vi "FileIoManager.vi"(8 "error in":errorcluster, 9 "slmDataSetIn":T1={"BeamParameters"={"amplitudeMatrix"=[], "SLM width (m)"=0.01536, "SLM height (m)"=0.00864, "wavelength (m)"=6.33e-07, "Resolution x"=1920, "Resolution y"=1080}, "BeamControl"={"xCenter"=0.0, "yCenter"=0.0, "xAngle_mRad"=4.5, "yAngle_mRad"=0.0, "beamWaist"=0.001}, "SLM Settings"={"resizeTo"=enum."Width of Display", "displayOn"=enum."All 2nd Monitor", "Top Left of Hologram"={"Horizontal"=80, "Vertical"=80}}, "Gamma Function"=245.0, "SLM colour coding"=enum."8-bit", "Masking?"=TRUE, "Calibration?"=FALSE, "Modes"=[{"type"=enum."LG Mode", "m or L"=2, "n or P"=0, "weight"=1.0, "phase"=0.0}, {"type"=enum."LG Mode", "m or L"=-2, "n or P"=0, "weight"=1.0, "phase"=0.0}, {"type"=enum."LG Mode", "m or L"=0, "n or P"=0, "weight"=0.0, "phase"=0.0}, {"type"=enum."LG Mode", "m or L"=0, "n or P"=0, "weight"=0.0, "phase"=0.0}], "Holo"=enum."Show", "BMP filePath"=path "C:/Users/science/Desktop/Filippo The 2nd/LabVIEW/Holos/SLMA/HG_2_2.bmp", "Power Meter Settings"={"Visa In"="", "Averaging Rate"=300, "Graph Length"=1000}, "Flip Image"=FALSE, "Mirror image"=FALSE, "Phase rotation"=0.0} {"Phase rotation" min=-6.2832 max=6.28318530718 step=0.01570796326; "BeamParameters"."Resolution y" format="%#.4g"; "BeamParameters"."Resolution x" format="%#.6g"}, 10 "file (use dialog)":path, 11 "state":enum16{"read", "write"}(ring)) -> (0 "error out":errorcluster, 1 "slmDataSetOut":T1={"BeamParameters"={"amplitudeMatrix"=[], "SLM width (m)"=0.01536, "SLM height (m)"=0.00864, "wavelength (m)"=6.33e-07, "Resolution x"=1920, "Resolution y"=1080}, "BeamControl"={"xCenter"=0.0, "yCenter"=0.0, "xAngle_mRad"=4.5, "yAngle_mRad"=0.0, "beamWaist"=0.001}, "SLM Settings"={"resizeTo"=enum."Width of Display", "displayOn"=enum."All 2nd Monitor", "Top Left of Hologram"={"Horizontal"=80, "Vertical"=80}}, "Gamma Function"=245.0, "SLM colour coding"=enum."8-bit", "Masking?"=TRUE, "Calibration?"=FALSE, "Modes"=[{"type"=enum."LG Mode", "m or L"=2, "n or P"=0, "weight"=1.0, "phase"=0.0}, {"type"=enum."LG Mode", "m or L"=-2, "n or P"=0, "weight"=1.0, "phase"=0.0}, {"type"=enum."LG Mode", "m or L"=0, "n or P"=0, "weight"=0.0, "phase"=0.0}, {"type"=enum."LG Mode", "m or L"=0, "n or P"=0, "weight"=0.0, "phase"=0.0}], "Holo"=enum."Show", "BMP filePath"=path "C:/Users/science/Desktop/Filippo The 2nd/LabVIEW/Holos/SLMA/HG_2_2.bmp", "Power Meter Settings"={"Visa In"="", "Averaging Rate"=300, "Graph Length"=1000}, "Flip Image"=FALSE, "Mirror image"=FALSE, "Phase rotation"=0.0} {"Phase rotation" min=-6.2832 max=6.28318530718 step=0.01570796326; "BeamParameters"."Resolution y" format="%#.4g"; "BeamParameters"."Resolution x" format="%#.6g"})   [LabVIEW 2020]
uses:
  typeDefs/fileIO.ctl
  typeDefs/BPandSLM.ctl
  typeDefs/beamData.ctl
  typeDefs/slmSettings.ctl
  typeDefs/modesArray.ctl
  typeDefs/modeCluster.ctl
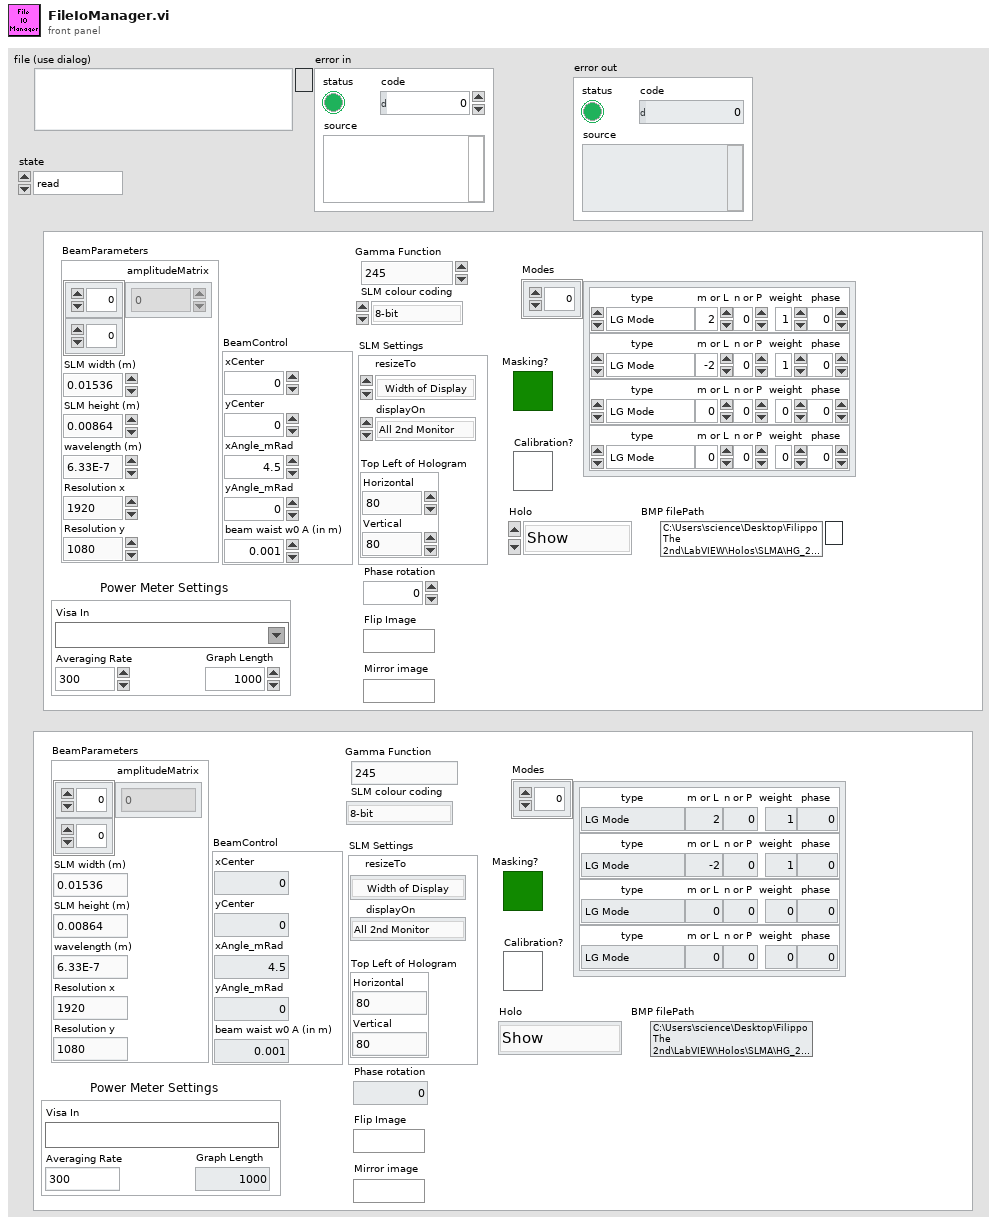
[diagram p1: front panel]
types:
  T1 = typedef "fileIO.ctl" = cluster{"BeamParameters":T2, "BeamControl":T3, "SLM Settings":T4, "Gamma Function":dbl, "SLM colour coding":enum16{"8-bit", "10-bit (Santec)"}, "Masking?":bool, "Calibration?":bool, "Modes":T5, "Holo":enum16{"Show", "Save BMP"}, "BMP filePath":path, "Power Meter Settings":cluster{"Visa In":refnum<visa-resource-name>, "Averaging Rate":i32, "Graph Length":i32}, "Flip Image":bool, "Mirror image":bool, "Phase rotation":dbl}
  T2 = typedef "BPandSLM.ctl" = cluster{"amplitudeMatrix":csg[][], "SLM width (m)":dbl, "SLM height (m)":dbl, "wavelength (m)":dbl, "Resolution x":u32, "Resolution y":u32}
  T3 = typedef "beamData.ctl" = cluster{"xCenter":dbl, "yCenter":dbl, "xAngle_mRad":dbl, "yAngle_mRad":dbl, "beamWaist":dbl}
  T4 = typedef "slmSettings.ctl" = cluster{"resizeTo":enum16{"No Resize", "Width of Display", "Height of Display"}, "displayOn":enum16{"Default", "All 1st Monitor", "All 2nd Monitor", "All 3rd Monitor", "All 4th Monitor"}, "Top Left of Hologram":cluster{"Horizontal":i16, "Vertical":i16}}
  T5 = typedef "modesArray.ctl" = T6[]
  T6 = typedef "modeCluster.ctl" = cluster{"type":enum16{"Azimuth Mode", "LG Mode", "HG Mode"}, "m or L":i32, "n or P":i32, "weight":dbl, "phase":dbl}
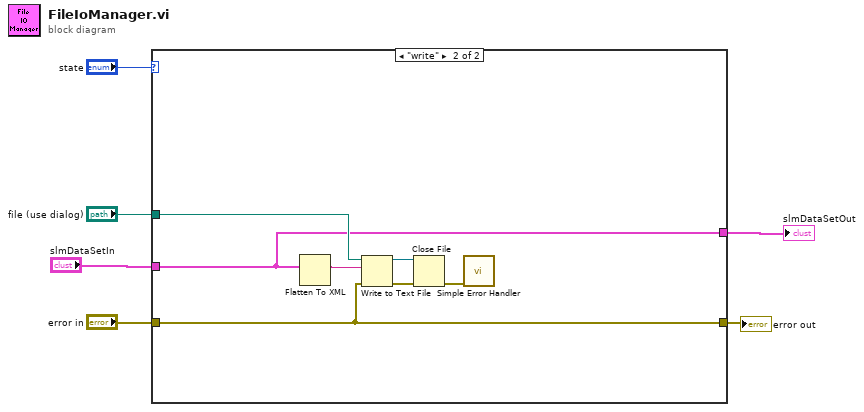
[diagram p0: block diagram]
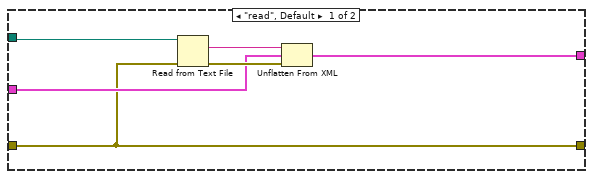
[diagram p2: hidden frame]
diagram:
  n1 = case shown="\"write\"" "state" {
    tunnel: "file (use dialog)" -> [w12 w18]
    tunnel: "error in" -> [w7 w14]
    tunnel: [w7 w14] -> w3
    tunnel: "slmDataSetIn" -> [w9 w13]
    tunnel: [w8 w13] -> w2
    frame "read", Default {
      n2 = Read from Text File(file (use dialog)=w12, error in=w7) -> (text=w11:string, error out=w10:errorcluster)  [unwired: 2 in, 2 out]
      n3 = Unflatten From XML(xml string=w11, type=w9, error in (no error)=w10) -> (value=w8:T1)  [unwired: 1 out]
    }
    frame "write" {
      n4 = Flatten To XML(6:w13) -> (2:w19:string)
      n5 = Write to Text File(file (use dialog)=w18, text=w19, error in=w14) -> (refnum out=w16:refnum<file>, error out=w17:errorcluster)  [unwired: 1 in, 1 out]
      n6 = Close File(refnum=w16, error in=w17) -> (error out=w15:errorcluster)  [unwired: 1 out]
      n7 = call <vilib>:"Simple Error Handler.vi"("error in (no error)"=w15) -> ()  [unwired: 4 in, 5 out]
    }
  }
  "error out" <- w3
  "slmDataSetOut" <- w2
